vi "sub_config_load-save.vi"(7 "cmd":enum16{"save", "load"}(ring)) -> (0 "error out":errorcluster)   [LabVIEW 2019]
uses:
  Breakdown-Spec.ctl
  Register/Setting_reg.ctl
  _ctrl/config_aging.ctl
  Register/Global_params_reg.vi
panel:
  in  "path":path
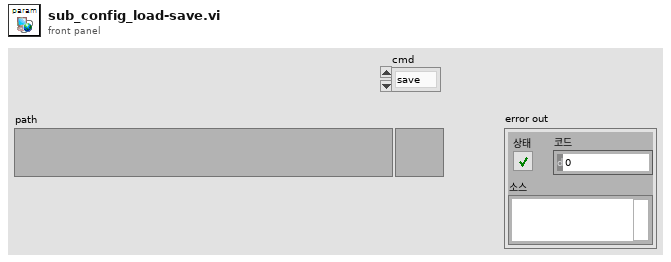
[diagram p1: front panel]
types:
  T1 = enum16{"open", "replace", "create", "open or create", "replace or create", "replace or create with confirmation"}
  T2 = typedef "config_aging.ctl" = cluster{"CapTest Config":T3, "TestName":string, "Result path":path, "파일 생성 주기[N]":dbl, "CapTest Specs":T4}
  T3 = typedef "Setting_reg.ctl" = cluster{"제어 전압[V]":dbl, "출력전압[V]":dbl, "전류[A]":dbl, "출력전류[A]":dbl, "ON[초]":dbl, "OFF[초]":dbl, "시험횟수[N]":u32, "Irms 허용치 from ":dbl, "Irms 허용치 to":dbl, "Ch selection":cluster{"ch 1":bool, "ch 2":bool, "ch 3":bool, "ch 4":bool, "ch 5":bool, "ch 6":bool}, "AO Delay ms":u32}
  T4 = typedef "Breakdown-Spec.ctl" = cluster{"제어단 단선 전류 RMS Max":dbl, "제어단 단락 전류 RMS Min":dbl, "제어단 특성 전류 RMS Max":dbl, "제어단 특성 전류 RMS Min":dbl, "출력단 전류 RMS Max":dbl, "출력단 전류 RMS Min":dbl, "출력단 특성 전류 RMS Max":dbl, "출력단 특성전류 RMS Min":dbl, "부하전압 RMS[+/-%] ":dbl, "온도[degree]":dbl}
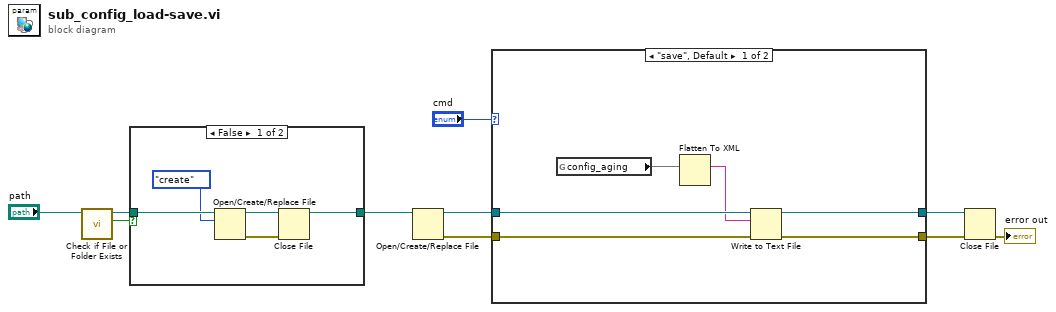
[diagram p0: block diagram]
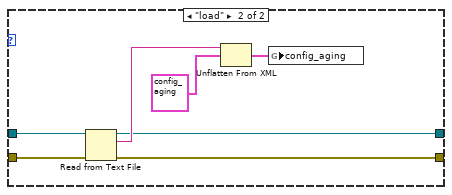
[diagram p3: hidden frame]
diagram:
  n1 = call <vilib>:"Check if File or Folder Exists.vi"("path"="path") -> ("file or folder exists?"=w4:bool, "dup path"=w2:path)  [unwired: 8 in, 1 out]
  n2 = case shown="False" w4 {
    tunnel: [w12 w16] -> w3
    tunnel: w2 -> [w15 w16]
    frame False {
      n3 = Open/Create/Replace File(file path (use dialog)=w15, operation (0:open)=T1."create" ("동작(0:open)")) -> (refnum out=w13:refnum<file>, error out=w11:errorcluster)  [unwired: 4 in, 1 out]
      n4 = Close File(refnum=w13, error in=w11) -> (path=w12:path)  [unwired: 1 out]
    }
    frame True {
    }
  }
  n5 = Open/Create/Replace File(file path (use dialog)=w3) -> (refnum out=w6:refnum<file>, error out=w7:errorcluster)  [unwired: 5 in, 1 out]
  n6 = case shown="\"save\", Default" "cmd" {
    tunnel: w6 -> [w19 w23]
    tunnel: [w21 w26] -> w9
    tunnel: [w20 w25] -> w8
    tunnel: w7 -> [w18 w24]
    frame "save", Default {
      n7 = global read "Global_params_reg.vi" "config_aging"() -> (w22)
      n8 = Flatten To XML(anything=w22) -> (xml string=w17:string)
      n9 = Write to Text File(file (use dialog)=w19, text=w17, error in=w18) -> (refnum out=w20:refnum<file>, error out=w21:errorcluster)  [unwired: 1 in, 1 out]
    }
    frame "load" {
      n10 = Read from Text File(file (use dialog)=w23, error in=w24) -> (refnum out=w25:refnum<file>, text=w29:string, error out=w26:errorcluster)  [unwired: 2 in, 1 out]
      n11 = Unflatten From XML(xml string=w29, type=T2 {"CapTest Config"={"제어 전압[V]"=0.0, "출력전압[V]"=0.0, "전류[A]"=0.0, "출력전류[A]"=0.0, "ON[초]"=0.0, "OFF[초]"=0.0, "시험횟수[N]"=100, "Irms 허용치 from "=0.0, "Irms 허용치 to"=0.0, "Ch selection"={"ch 1"=TRUE, "ch 2"=TRUE, "ch 3"=FALSE, "ch 4"=FALSE, "ch 5"=TRUE, "ch 6"=FALSE}, "AO Delay ms"=0}, "TestName"="", "Result path"=path "", "파일 생성 주기[N]"=0.0, "CapTest Specs"={"제어단 단선 전류 RMS Max"=0.0, "제어단 단락 전류 RMS Min"=0.0, "제어단 특성 전류 RMS Max"=0.0, "제어단 특성 전류 RMS Min"=0.0, "출력단 전류 RMS Max"=0.0, "출력단 전류 RMS Min"=0.0, "출력단 특성 전류 RMS Max"=0.0, "출력단 특성전류 RMS Min"=0.0, "부하전압 RMS[+/-%] "=0.0, "온도[degree]"=0.0}} ("config_aging")) -> (value=w27:T2)  [unwired: 1 in, 1 out]
      n12 = global write "Global_params_reg.vi" "config_aging"(w27) -> ()
    }
  }
  n13 = Close File(refnum=w8, error in=w9) -> (error out=→"error out":errorcluster)  [unwired: 1 out]
